vi "CloneManyMethods.vi"(1 "VIRefs":refnum<vi>[](array[refnum]), 5 "error in (no error)":errorcluster) -> (17 "Cancelled":bool, 19 "error out":errorcluster)   [LabVIEW 2020]
uses:
  <resource>/Framework/Providers/Open_GDS/SubVIs/GOOP_HelpButton.ctl
  <vilib>/picture/picture.llb/imagedata.ctl
  <vilib>/Utility/lvfile.llb/NI_FileType.lvlib
  <resource>/Framework/Providers/Open_GDS/ClassProviders/Provider_LvNativeClass/ClassWriterNative_class/ClassWriterNative.lvclass
panel:
  out "ProductPicture":picture
  in  "_CloneAndOpenVI":bool
  in  "_OverwirteTragetVIs":bool
  in  "_CloneMethodClasses":i32[](listbox) caption="Select which classes to clone the VI to"
  out "_ViPathAlreadyExists":bool=TRUE caption="This VI already exists"
  out "_CloneViName":string caption="Original VI Name"
  in  "_ClassOwner":u16(ring) caption="New VI Owner" items=["<Clone VIs to Selected Sibling Classes>", "<Clone VIs to Selected Classes>"]
  in  "_HelpCloneClass":T1
  in  "_Cancel":bool
  in  "_CloneVI":bool
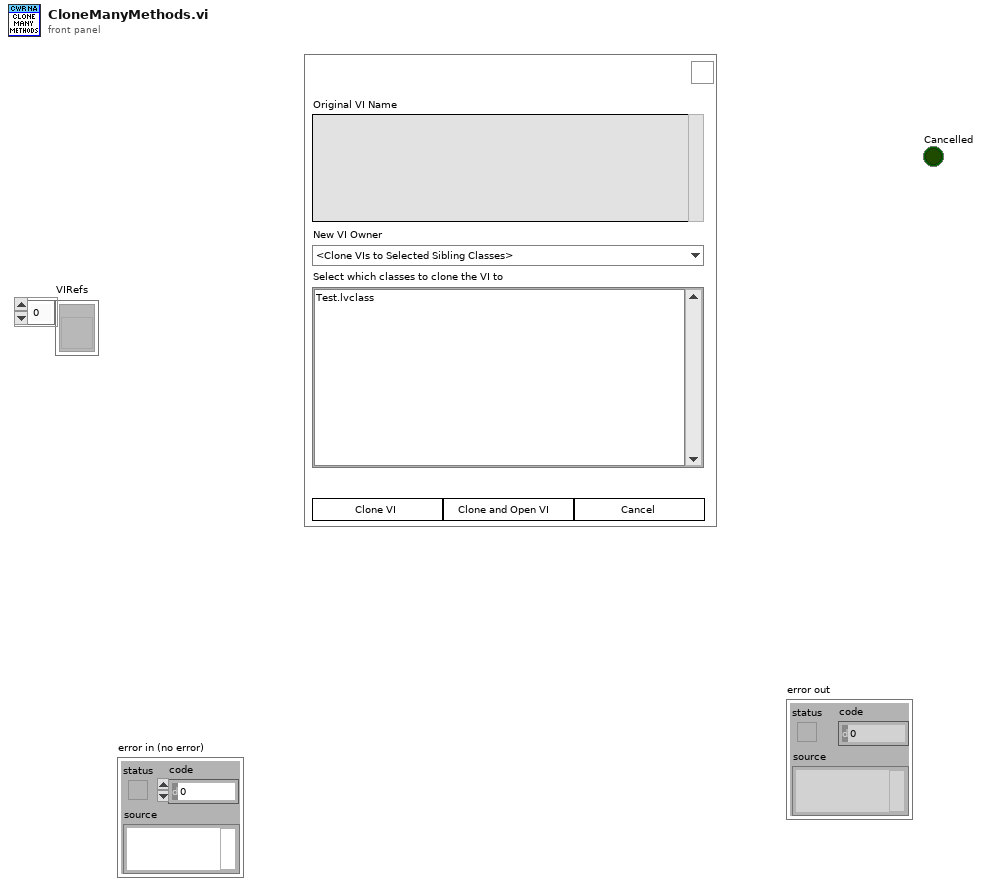
[diagram p1: front panel]
types:
  T1 = typedef "GOOP_HelpButton.ctl" = bool
  T2 = cluster{"Cancel":bool, "OrgVIPath":path, "Libs":refnum<vi>[], "SiblingClasses":refnum<vi>[], "ProjectFolder":path, "ViRelFromParent":path, "ManyClasses":bool, "OrgLibName":string, "AllClasses":refnum<vi>[], "OpenAfter":bool, "VIName":string[], "VIExt":string[], "AppRef":refnum<vi>, "VIOwner":refnum<vi>, "OrgViLibName":string, "OrgLibFolder":path, "OrgClassPath":path, "OrgClassPathMemberData":path, "FileBackups":string[], "CopyToTheseClasses":refnum<vi>[], "VIRef":refnum<vi>[], "OrgPath":path[], "Scope":enum32{"invalid scope", "public", "private", "protected", "community"}[], "NewViRefs":cluster{refnum<vi>[]}[], "NewVIPaths":path[]}
  T3 = enum32{"invalid scope", "public", "private", "protected", "community"}
  T4 = typedef "imagedata.ctl" = cluster{"image type":i32, "image depth":i32, "image":u8[], "mask":u8[], "colors":u32[], "Rectangle":cluster{"left":i16, "top":i16, "right":i16, "bottom":i16}}
  T5 = enum32{"invalid scope", "public", "private", "protected", "community"}[]
  T6 = typedef "GDSLvClass_IconSettingsType.ctl" = cluster{"Frame":u32, "Frame thickness":u8, "Header Background":u32, "Header Text":u32, "ColorPublic":u32, "ColorProtected":u32, "ColorPrivate":u32, "Body Text":u32, "ClassBodyIcon":string}
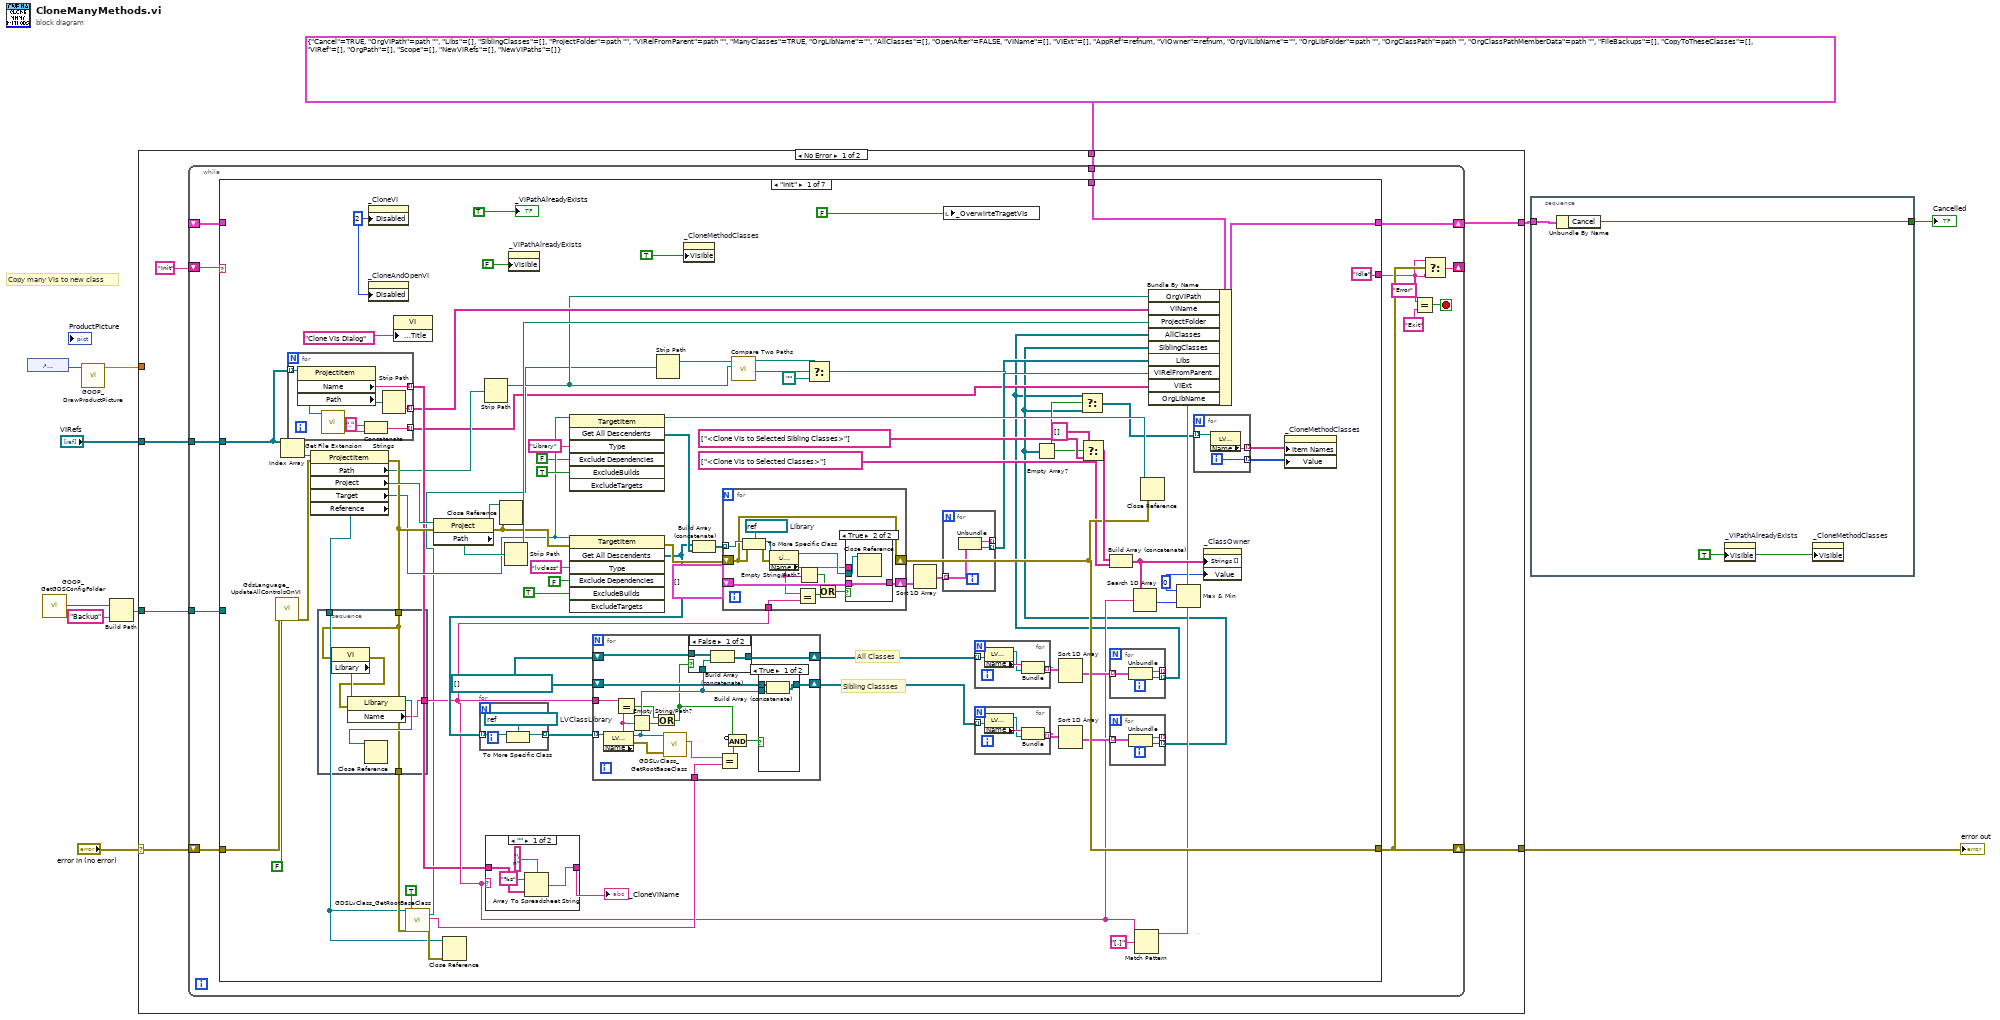
[diagram p0: block diagram]
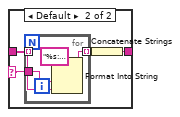
[diagram p2: hidden frame]
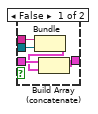
[diagram p5: hidden frame]
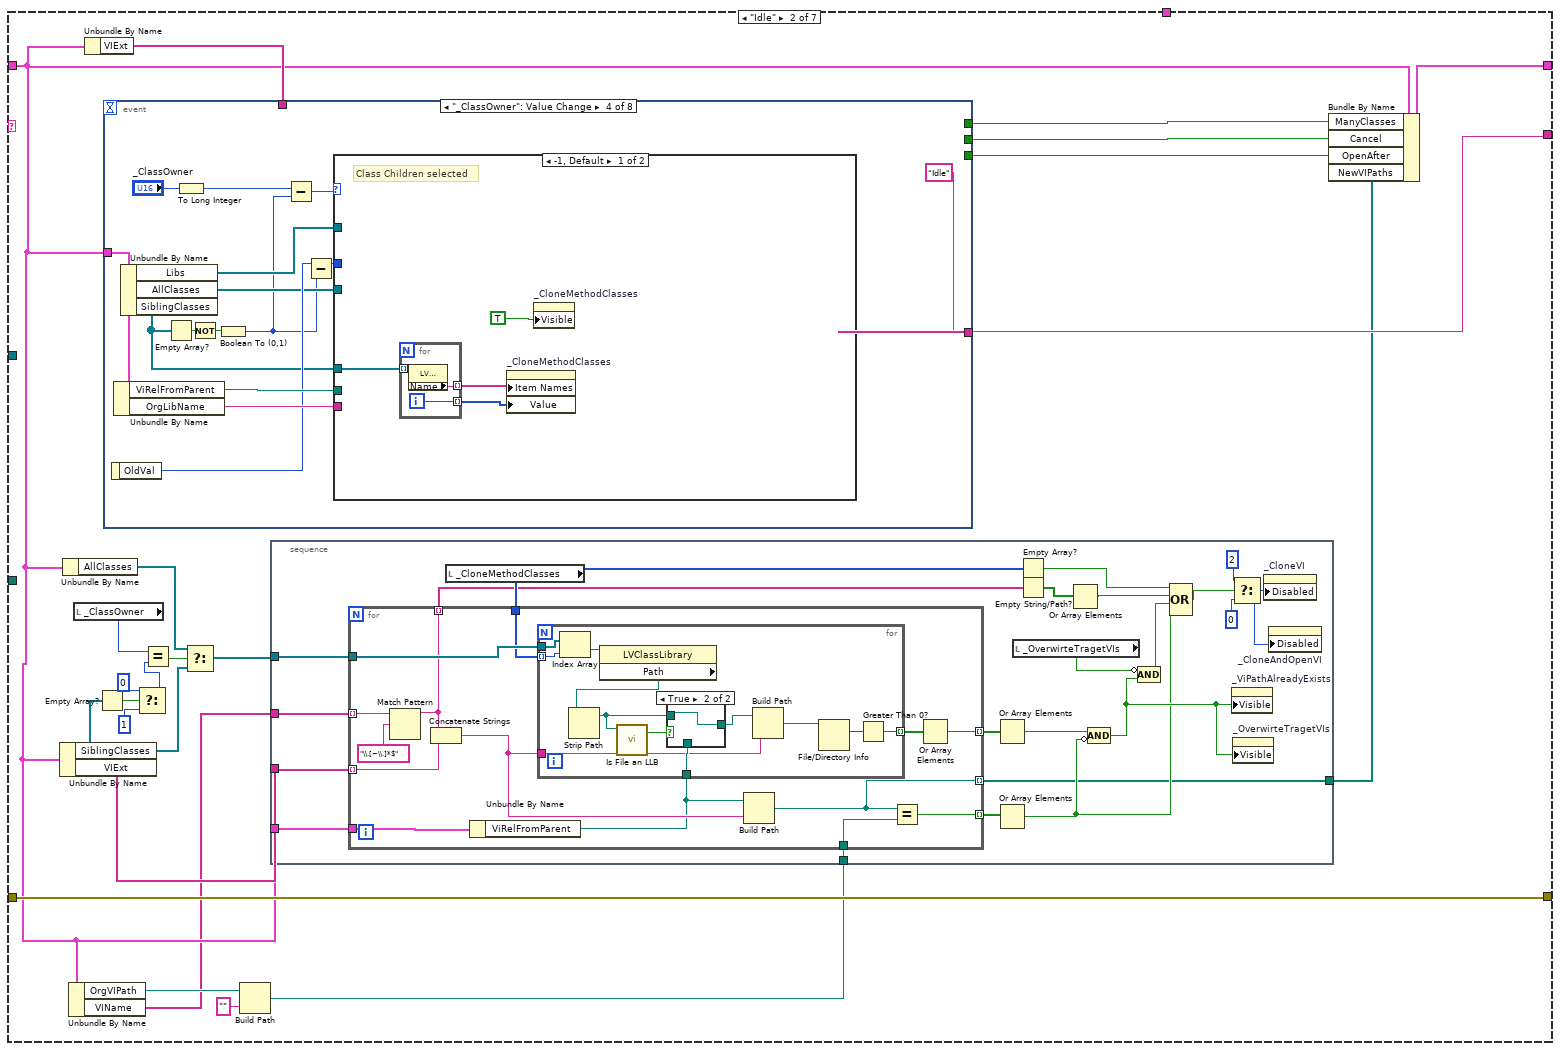
[diagram p6: hidden frame]
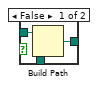
[diagram p7: hidden frame]
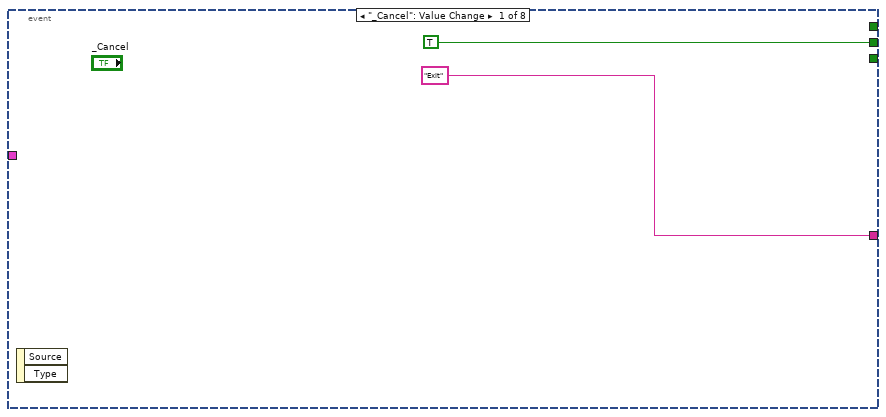
[diagram p8: hidden frame]
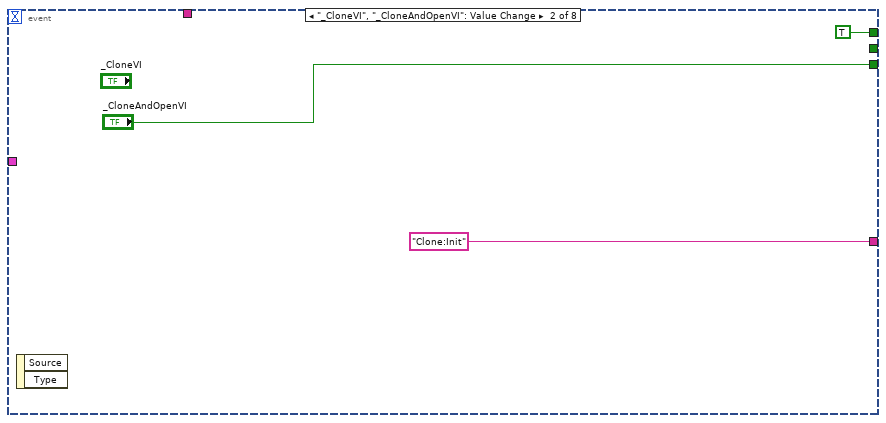
[diagram p9: hidden frame]
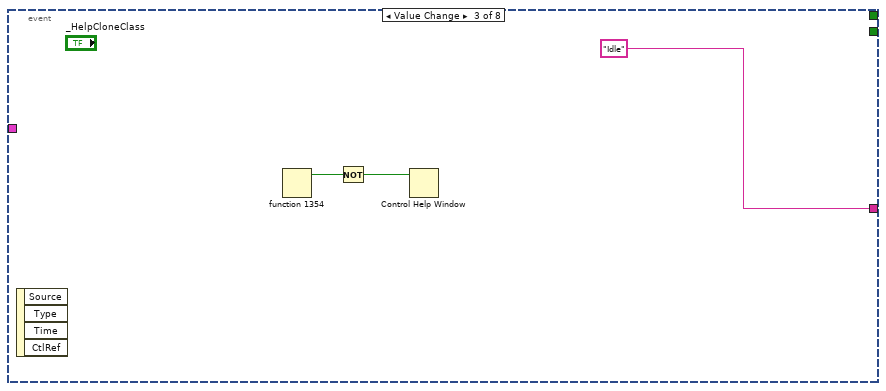
[diagram p10: hidden frame]
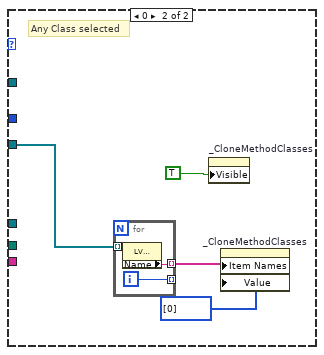
[diagram p11: hidden frame]
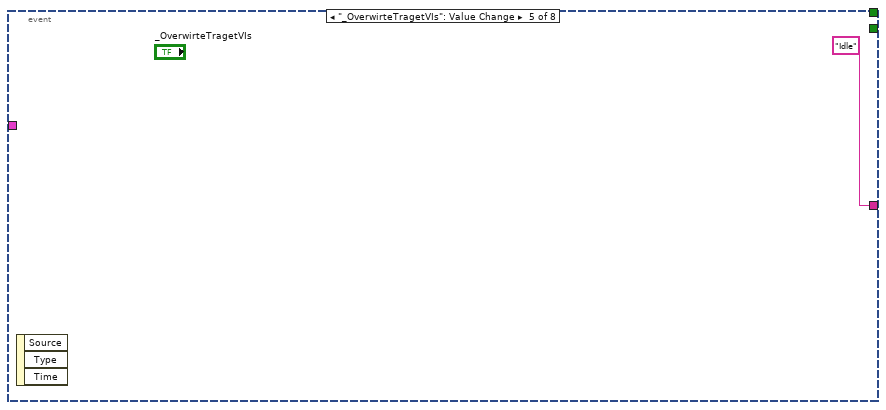
[diagram p12: hidden frame]
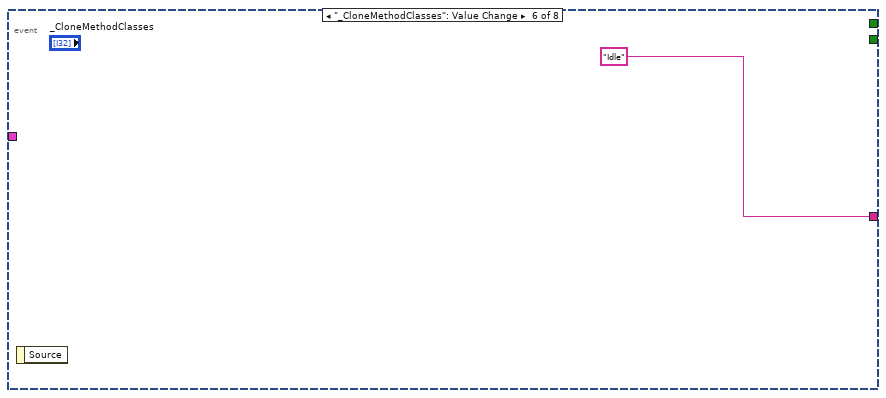
[diagram p13: hidden frame]
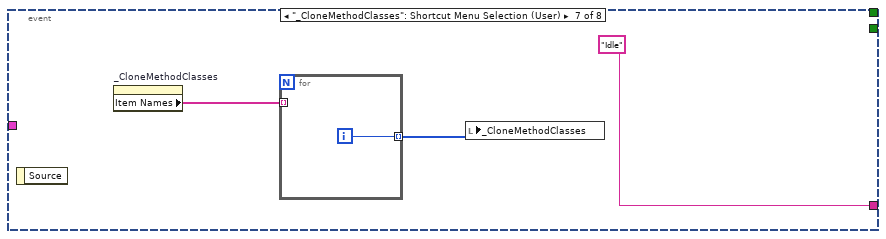
[diagram p14: hidden frame]
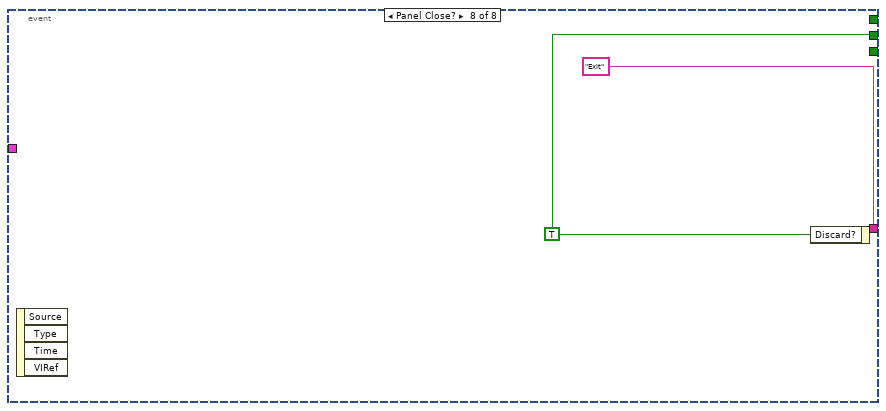
[diagram p15: hidden frame]
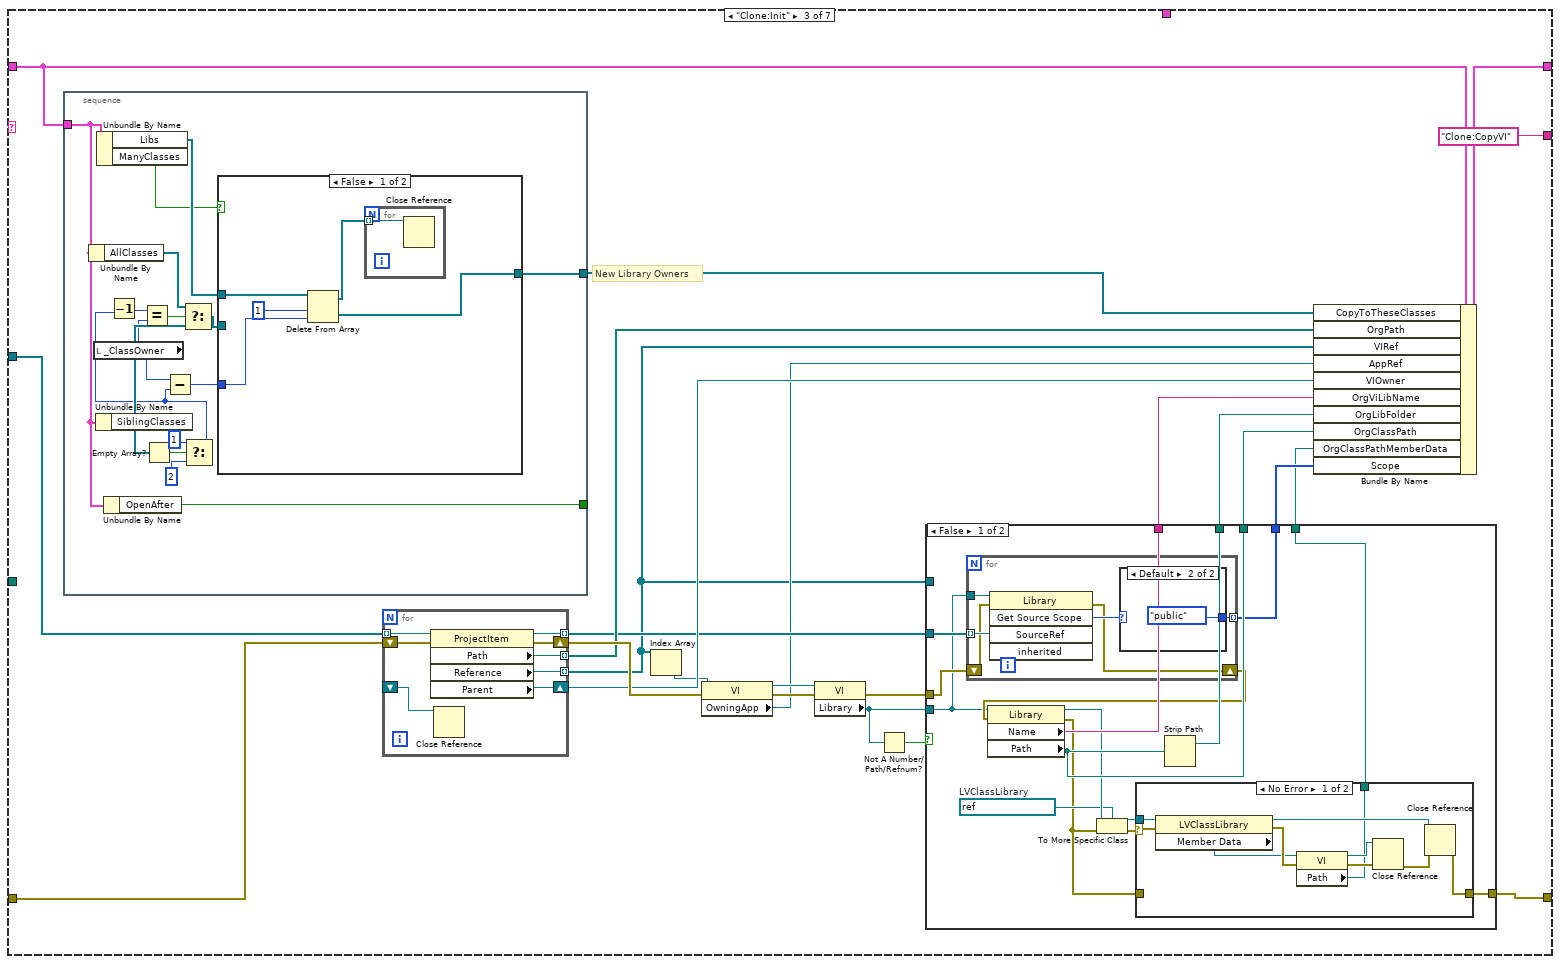
[diagram p16: hidden frame]
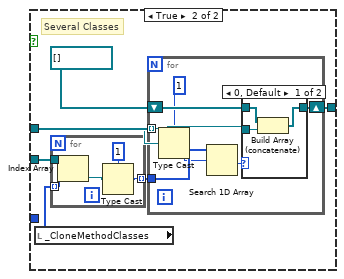
[diagram p17: hidden frame]
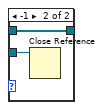
[diagram p18: hidden frame]
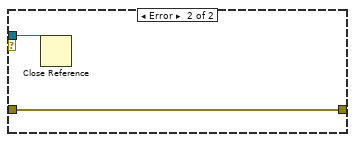
[diagram p20: hidden frame]
diagram:
  # "Copy many VIs to new class"
  n1 = control-ref of="ProductPicture"() -> (w2:refnum<vi>)
  n2 = call <resource>:"GOOP_GetGDSConfigFolder.vi"() -> ("GDSFolderPath"=w4:path)
  n3 = call <resource>:"GOOP_DrawProductPicture.vi"("ProductPictureControl"=w2) -> ("Zoom Factor"=w1:sgl)  [unwired: 10 in]
  n4 = Build Path(base path=w4, name or relative path="Backup") -> (appended path=w3:path)
  n5 = case shown="No Error" "error in (no error)" {
    selector: "error in (no error)" -> [w18 w819]
    tunnel: [w17 w819] -> w8
    tunnel: T2 {"Cancel"=TRUE, "OrgVIPath"=path "", "Libs"=[], "SiblingClasses"=[], "ProjectFolder"=path "", "ViRelFromParent"=path "", "ManyClasses"=TRUE, "OrgLibName"="", "AllClasses"=[], "OpenAfter"=FALSE, "VIName"=[], "VIExt"=[], "AppRef"=refnum, "VIOwner"=refnum, "OrgViLibName"="", "OrgLibFolder"=path "", "OrgClassPath"=path "", "OrgClassPathMemberData"=path "", "FileBackups"=[], "CopyToTheseClasses"=[], "VIRef"=[], "OrgPath"=[], "Scope"=[], "NewViRefs"=[], "NewVIPaths"=[]} ("output cluster") -> [w16 _]
    tunnel: "VIRefs" -> [w15 _]
    tunnel: [w14 _] -> w10
    tunnel: w3 -> [w12 _]
    tunnel: w1 -> [_ _]
    frame No Error {
      n6 = while {
        shift-right: [w25] -> w17
        shift-left: w18 -> [w31]
        shift-right: [w24] -> _
        shift-left: "Init" -> [w28]
        shift-right: [w29] -> w14
        shift-left: _ -> [w30]
        tunnel: w16 -> [w21]
        tunnel: w15 -> [w20]
        tunnel: w12 -> [w19]
        stop <- w26 stop-if-true
        n7 = case shown="\"Init\"" w28 {
          tunnel: w30 -> [_ w207 w326 w445 w620 w660 w769]
          tunnel: [w108 w222 w328 w447 w620 w660 w769] -> w29
          tunnel: w31 -> [w106 w224 w329 w449 w623 w663 w772]
          tunnel: [w79 w224 w330 w448 w622 w662 w771] -> w25
          tunnel: ["Idle" w223 "Clone:CopyVI" w446 "Clone:UpdateIcon" "Done" "Exit"] -> w23
          tunnel: w21 -> [w107 _ _ _ _ _ _]
          tunnel: w20 -> [w44 _ w324 _ _ _ _]
          tunnel: w19 -> [_ _ _ w443 _ _ w770]
          frame "Init" {
            w51 = 0 ("Text.Selection:Start")
            w73 = refnum<vi>[] []
            w71 = u8 2 ("Disabled")
            # "Sibling Classses"
            # "All Classes"
            n8 = call <resource>:"GdsLanguage_UpdateAllControlsOnVI.vi"("error in (no error)"=w106, "CreateLanguageFile(Use this to create a languageFile)"=FALSE) -> ("error out"=w52:errorcluster)  [unwired: 16 in, 1 out]
            n9 = Index Array(array=w44) -> (element=w45:refnum<vi>)  [unwired: 1 in]
            n10 = for {
              tunnel: w44 -> [w119] mode=indexing
              tunnel: [w118] -> w48 mode=indexing
              tunnel: [w117] -> w47 mode=indexing
              tunnel: [w113] -> w41 mode=indexing
              n11 = property class="ProjectItem"(reference=w119) -> ("Name"=w118:string, "Path"=w116:path)  [unwired: 1 in, 2 out]
              n12 = call <vilib>:"Get File Extension.vi"("file"=w116) -> ("lowercase file extension"=w114:string)  [unwired: 6 in, 4 out]
              n13 = Concatenate Strings("." ("string"), w114) -> (w113:string)
              n14 = Strip Path(path=w116) -> (name=w117:string)  [unwired: 1 out]
            }
            n15 = property class="ProjectItem"(reference=w45, error in=w52) -> (error out=w59:errorcluster, "Path"=w46:path, "Project"=w103:refnum<vi>, "Target"=w53:refnum<vi>, "Reference"=w54:refnum<vi>)  [unwired: 1 out]
            n16 = stacked-sequence {
              tunnel: w54 -> [w125]
              tunnel: w59 -> [w121]
              tunnel: [w120] -> w50
              tunnel: [w121] -> w58
              frame #0 {
                n17 = property class="VI"(reference=w125, error in=w121) -> (error out=w123:errorcluster, "Library"=w124:refnum<vi>)  [unwired: 1 out]
                n18 = property class="Library"(reference=w124, error in=w123) -> (reference out=w122:refnum<vi>, "Name"=w120:string)  [unwired: 1 out]
                n19 = Close Reference(reference=w122) -> ()  [unwired: 1 in, 1 out]
              }
            }
            n20 = property on="_CloneVI" class="Bool"("Disabled"=w71) -> ()  [unwired: 2 in, 2 out]
            n21 = property on="_CloneAndOpenVI" class="Bool"("Disabled"=w71) -> ()  [unwired: 2 in, 2 out]
            n22 = property class="VI"("Front Panel.Title"="Clone VIs Dialog" ("format string")) -> ()  [unwired: 2 in, 2 out]
            n23 = call <resource>:"GDSLvClass_GetRootBaseClass.vi"("ViRef/Path,LvClassRef/Path"=w54, "error in (no error)"=w58, "Don'tOpenReference"=TRUE) -> ("RootBaseClassPath"=w42:path, "ClassName"=w67:string, "error out"=w68:errorcluster)  [unwired: 10 in, 4 out]
            n24 = property class="Project"(reference=w103, error in=w59) -> (reference out=w80:refnum<vi>, error out=w81:errorcluster, "Path"=w83:path)
            n25 = Close Reference(reference=w54, error in (no error)=w68) -> ()  [unwired: 1 out]
            n26 = Strip Path(path=w46) -> (stripped path=w43:path)  [unwired: 1 out]
            n27 = case shown="\"\"" w50 {
              selector: w50 -> [_ w148]
              tunnel: w48 -> [w144 w150]
              tunnel: [w143 w147] -> w82
              frame "" {
                n28 = Array To Spreadsheet String(delimiter (Tab)="\n", array=w144, 3:"%s" ("format string")) -> (spreadsheet string=w143:string)
              }
              frame Default {
                n29 = for {
                  tunnel: w150 -> [w153] mode=indexing
                  tunnel: [w152] -> w149 mode=indexing
                  tunnel: w148 -> [w151]
                  n30 = Format Into String(format string="%s:%s\n", w151, w153) -> (resulting string=w152:string)  [unwired: 2 in, 1 out]
                }
                n31 = Concatenate Strings(w149) -> (w147:string)
              }
            }
            "_CloneViName" <- w82
            n32 = Close Reference(reference=w80, error in (no error)=w81) -> ()  [unwired: 1 out]
            n33 = Strip Path(path=w83) -> (stripped path=w88:path)  [unwired: 1 out]
            n34 = property on="_ViPathAlreadyExists" class="Bool (strict)"("Visible"=FALSE) -> ()  [unwired: 2 in, 2 out]
            n35 = invoke class="TargetItem" method="Get All Descendents"(reference=w53, "Type"="Library", "Exclude Dependencies"=FALSE ("ExcludeDependencies"), "ExcludeBuilds"=TRUE ("ExcludeDependencies")) -> (reference out=w78:refnum<vi>, "All Descendents"=w96:refnum<vi>[])  [unwired: 3 in, 5 out]
            n36 = invoke class="TargetItem" method="Get All Descendents"(reference=w53, error in=w81, "Type"="lvclass", "Exclude Dependencies"=FALSE ("ExcludeDependencies"), "ExcludeBuilds"=TRUE ("ExcludeDependencies")) -> (error out=w101:errorcluster, "All Descendents"=w94:refnum<vi>[])  [unwired: 2 in, 5 out]
            n37 = for {
              tunnel: w94 -> [w156] mode=indexing
              tunnel: [w155] -> w72 mode=indexing
              w157 = refnum<vi> refnum  # LVClassLibrary
              n38 = To More Specific Class(target class=w157, reference=w156) -> (specific class reference=w155:refnum<vi>)  [unwired: 1 in, 1 out]
            }
            n39 = for {
              tunnel: w72 -> [w173] mode=indexing
              tunnel: w67 -> [w165]
              shift-right: [w171] -> w60
              shift-left: w73 -> [w172]
              shift-right: [w169] -> w63
              shift-left: w73 -> [w170]
              tunnel: w50 -> [w168]
              n40 = property class="LVClassLibrary"(reference=w173) -> (reference out=w167:refnum<vi>, error out=w166:errorcluster, "Name"=w161:string)  [unwired: 1 in]
              n41 = Equal?(x=w168, y=w161) -> (x = y?=w159:bool)
              n42 = Empty String/Path?(string/path=w161) -> (empty?=w160:bool)
              n43 = Or(x=w159, y=w160) -> (x .or. y?=w158:bool)
              n44 = call <resource>:"GDSLvClass_GetRootBaseClass.vi"("ViRef/Path,LvClassRef/Path"=w167, "error in (no error)"=w166) -> ("ClassName"=w164:string)  [unwired: 11 in, 6 out]
              n45 = case shown="False" w158 {
                tunnel: w170 -> [w176 w177]
                tunnel: w167 -> [w175 _]
                tunnel: [w174 w177] -> w169
                frame False {
                  n46 = Build Array (concatenate)(w176, w175) -> (w174:refnum<vi>[])
                }
                frame True {
                }
              }
              n47 = Equal?(x=w164, y=w165) -> (x = y?=w163:bool)
              n48 = Compound Arithmetic op=AND(invert w158, w163) -> (w162:bool)
              n49 = case shown="True" w162 {
                tunnel: w172 -> [w180 w181]
                tunnel: w167 -> [w179 _]
                tunnel: [w178 w181] -> w171
                frame True {
                  n50 = Build Array (concatenate)(w180, w179) -> (w178:refnum<vi>[])
                }
                frame False {
                }
              }
            }
            n51 = Strip Path(path=w42) -> (stripped path=w89:path)  [unwired: 1 out]
            n52 = property on="_CloneMethodClasses" class="LstBox (strict)"("Visible"=TRUE) -> ()  [unwired: 2 in, 2 out]
            n53 = Build Array (concatenate)(w94, w96) -> (w95:refnum<vi>[])
            n54 = for {
              tunnel: w95 -> [w194] mode=indexing
              shift-right: [w189] -> w79
              shift-left: w101 -> [w189]
              shift-right: [w187] -> w56
              shift-left: cluster{"Name":string, refnum<vi>}[] [] -> [w188]
              tunnel: w50 -> [w186]
              w192 = refnum<vi> refnum  # Library
              n55 = To More Specific Class(target class=w192, reference=w194, error in=w189) -> (specific class reference=w193:refnum<vi>, error out=w191:errorcluster)
              n56 = property class="Library"(reference=w193, error in=w191) -> (reference out=w190:refnum<vi>, "Name"=w182:string)  [unwired: 1 out]
              n57 = Equal?(x=w182, y=w186) -> (x = y?=w184:bool)
              n58 = Empty String/Path?(string/path=w182) -> (empty?=w185:bool)
              n59 = Or(x=w185, y=w184) -> (x .or. y?=w183:bool)
              n60 = case shown="True" w183 {
                tunnel: w182 -> [w199 _]
                tunnel: w190 -> [w198 w200]
                tunnel: w188 -> [w197 w201]
                tunnel: [w195 w201] -> w187
                frame False {
                  n61 = Bundle("Name"=w199, w198) -> (w196:cluster{"Name":string, refnum<vi>})  [unwired: 1 in]
                  n62 = Build Array (concatenate)(w197, w196) -> (w195:cluster{"Name":string, refnum<vi>}[])
                }
                frame True {
                  n63 = Close Reference(reference=w200) -> ()  [unwired: 1 in, 1 out]
                }
              }
            }
            n64 = call <vilib>:"Compare Two Paths.vi"("Path 2"=w43, "Path 1"=w89) -> ("Path 2 Relative to Path 1?"=w87:bool, "Relative Path from 1 to 2"=w86:path)  [unwired: 6 in, 2 out]
            n65 = Select(t=w86, s=w87, f=path "") -> (s? t:f=w84:path)
            n66 = Sort 1D Array(array=w56) -> (sorted array=w70:cluster{"Name":string, refnum<vi>}[])
            n67 = for {
              tunnel: w70 -> [w142] mode=indexing
              tunnel: [w141] -> _ mode=indexing
              tunnel: [w140] -> w69 mode=indexing
              n68 = Unbundle(w142) -> ("Name"=w141:string, w140:refnum<vi>)
            }
            n69 = local write "_OverwirteTragetVIs"(FALSE ("Visible")) -> ()
            n70 = for {
              tunnel: w63 -> [w136] mode=indexing
              tunnel: [w137] -> w65 mode=indexing
              n71 = property class="LVClassLibrary"(reference=w136) -> (reference out=w138:refnum<vi>, "Name"=w139:string)  [unwired: 1 in, 1 out]
              n72 = Bundle("Name"=w139, w138) -> (w137:cluster{"Name":string, refnum<vi>})  [unwired: 1 in]
            }
            n73 = for {
              tunnel: w60 -> [w129] mode=indexing
              tunnel: [w130] -> w61 mode=indexing
              n74 = property class="LVClassLibrary"(reference=w129) -> (reference out=w131:refnum<vi>, "Name"=w132:string)  [unwired: 1 in, 1 out]
              n75 = Bundle("Name"=w132, w131) -> (w130:cluster{"Name":string, refnum<vi>})  [unwired: 1 in]
            }
            n76 = Sort 1D Array(array=w65) -> (sorted array=w64:cluster{"Name":string, refnum<vi>}[])
            n77 = Sort 1D Array(array=w61) -> (sorted array=w62:cluster{"Name":string, refnum<vi>}[])
            n78 = for {
              tunnel: w64 -> [w135] mode=indexing
              tunnel: [w134] -> _ mode=indexing
              tunnel: [w133] -> w35 mode=indexing
              n79 = Unbundle(w135) -> ("Name"=w134:string, w133:refnum<vi>)
            }
            n80 = for {
              tunnel: w62 -> [w128] mode=indexing
              tunnel: [w127] -> _ mode=indexing
              tunnel: [w126] -> w37 mode=indexing
              n81 = Unbundle(w128) -> ("Name"=w127:string, w126:refnum<vi>)
            }
            n82 = Empty Array?(array=w37) -> (empty?=w38:bool)
            n83 = Select(t=w35, s=w38, f=w37) -> (s? t:f=w36:refnum<vi>[])
            n84 = Select(t=string[] [], s=w38, f=string[] ["<Clone VIs to Selected Sibling Classes>"]) -> (s? t:f=w93:string[])
            n85 = Build Array (concatenate)(w93, string[] ["<Clone VIs to Selected Classes>"]) -> (w100:string[])
            n86 = Search 1D Array(1D array=w100, element=w50) -> (index of element=w99:i32)  [unwired: 1 in]
            n87 = Match Pattern(string=w50, regular expression="[.]") -> (before substring=w76:string)  [unwired: 1 in, 3 out]
            n88 = Close Reference(reference=w78, error in (no error)=w79) -> ()  [unwired: 1 out]
            n89 = Bundle By Name(cluster=w107, "OrgVIPath"=w43, "VIName"=w47, "ProjectFolder"=w88, "AllClasses"=w35, "SiblingClasses"=w37, "Libs"=w69, "ViRelFromParent"=w84, "VIExt"=w41, "OrgLibName"=w76) -> (w108:T2)
            n90 = Max & Min(x=w51, y=w99) -> ()  [unwired: 2 out]
            n91 = for {
              tunnel: [w112] -> w40 mode=indexing
              tunnel: w36 -> [w111] mode=indexing
              tunnel: [w110] -> w39 mode=indexing
              i -> [w110]
              n92 = property class="LVClassLibrary"(reference=w111) -> ("Name"=w112:string)  [unwired: 1 in, 2 out]
            }
            n93 = property on="_ClassOwner" class="Ring (strict)"("Strings []"=w100, "Value"=w51) -> ()  [unwired: 2 in, 2 out]
            n94 = property on="_CloneMethodClasses" class="LstBox (strict)"("Item Names"=w40, "Value"=w39) -> ()  [unwired: 2 in, 2 out]
            "_ViPathAlreadyExists" <- TRUE ("Visible")
          }
          frame "Idle" {
            n95 = Unbundle By Name(w207) -> ("SiblingClasses"=w213:refnum<vi>[], "VIExt"=w219:string[])
            n96 = Unbundle By Name(w207) -> ("AllClasses"=w216:refnum<vi>[])
            n97 = Unbundle By Name(w207) -> ("OrgVIPath"=w206:path, "VIName"=w204:string[])
            n98 = local read "_ClassOwner"() -> (w211:u16)
            n99 = Unbundle By Name(w207) -> ("VIExt"=w220:string[])
            n100 = Empty Array?(array=w213) -> (empty?=w214:bool)
            n101 = event shown="[3] \"_ClassOwner\": Value Change" {
              selector: _ -> [_ _ _ _ _ _ _ _]
              dyn-events: _ -> [_ _ _ _ _ _ _ _]
              timeout: _ -> [_ _ _ _ _ _ _ _]
              tunnel: ["Exit" "Clone:Init" "Idle" "Idle" "Idle" "Idle" "Idle" "Exit"] -> w223
              tunnel: [TRUE _ _ _ _ _ _ w321] -> w221
              tunnel: w207 -> [_ _ _ w296 _ _ _ _]
              tunnel: w220 -> [_ _ _ _ _ _ _ _]
              tunnel: [_ TRUE ("Visible") _ _ _ _ _ _] -> w218
              tunnel: [_ "_CloneAndOpenVI" _ _ _ _ _ _] -> w208
              event "_Cancel": Value Change {
                n102 = event-data() -> ()  [unwired: 1 in, 2 out]
              }
              event "_CloneVI", "_CloneAndOpenVI": Value Change {
                n103 = event-data() -> ()  [unwired: 1 in, 2 out]
              }
              event Value Change {
                n104 = event-data() -> ()  [unwired: 1 in, 4 out]
                n105 = fn#1354() -> (1:w284:bool)  [unwired: 1 out]
                n106 = Not(x=w284) -> (.not. x?=w283:bool)
                n107 = Control Help Window(1:w283) -> ()  [unwired: 1 in]
              }
              event "_ClassOwner": Value Change {
                n108 = event-data() -> ("OldVal"=w291:u16)  [unwired: 1 in]
                n109 = Unbundle By Name(w296) -> ("ViRelFromParent"=w295:path, "OrgLibName"=w292:string)
                n110 = Unbundle By Name(w296) -> ("Libs"=w297:refnum<vi>[], "AllClasses"=w288:refnum<vi>[], "SiblingClasses"=w289:refnum<vi>[])
                n111 = Empty Array?(array=w289) -> (empty?=w298:bool)
                n112 = To Long Integer(number="_ClassOwner") -> (32bit integer=w290:i32)
                n113 = Not(x=w298) -> (.not. x?=w293:bool)
                n114 = Boolean To (0,1)(Boolean=w293) -> (0, 1=w285:i16)
                n115 = Subtract(x=w290, y=w285) -> (x-y=w287:i32)
                n116 = Subtract(x=w291, y=w285) -> (x-y=w286:u16)
                n117 = case shown="-1, Default" w287 {
                  tunnel: w297 -> [_ _]
                  tunnel: w295 -> [_ _]
                  tunnel: w292 -> [_ _]
                  tunnel: w286 -> [_ _]
                  tunnel: w289 -> [w302 _]
                  tunnel: w288 -> [_ w308]
                  frame -1, Default {
                    # "Class Children selected"
                    n118 = for {
                      tunnel: [w306] -> w301 mode=indexing
                      tunnel: w302 -> [w305] mode=indexing
                      tunnel: [w304] -> w300 mode=indexing
                      i -> [w304]
                      n119 = property class="LVClassLibrary"(reference=w305) -> ("Name"=w306:string)  [unwired: 1 in, 2 out]
                    }
                    n120 = property on="_CloneMethodClasses" class="LstBox (strict)"("Item Names"=w301, "Value"=w300) -> ()  [unwired: 2 in, 2 out]
                    n121 = property on="_CloneMethodClasses" class="LstBox (strict)"("Visible"=TRUE) -> ()  [unwired: 2 in, 2 out]
                  }
                  frame 0 {
                    # "Any Class selected"
                    n122 = for {
                      tunnel: [w313] -> w309 mode=indexing
                      tunnel: w308 -> [w312] mode=indexing
                      tunnel: [w311] -> _ mode=indexing
                      i -> [w311]
                      n123 = property class="LVClassLibrary"(reference=w312) -> ("Name"=w313:string)  [unwired: 1 in, 2 out]
                    }
                    n124 = property on="_CloneMethodClasses" class="LstBox (strict)"("Visible"=TRUE) -> ()  [unwired: 2 in, 2 out]
                    n125 = property on="_CloneMethodClasses" class="LstBox (strict)"("Item Names"=w309, "Value"=i32[] [0] ("_CloneMethodClasses")) -> ()  [unwired: 2 in, 2 out]
                  }
                }
              }
              event "_OverwirteTragetVIs": Value Change {
                n126 = event-data() -> ()  [unwired: 1 in, 3 out]
              }
              event "_CloneMethodClasses": Value Change {
                n127 = event-data() -> ()  [unwired: 1 in, 1 out]
              }
              event "_CloneMethodClasses": Shortcut Menu Selection (User) {
                n128 = event-data() -> ()  [unwired: 1 in, 1 out]
                n129 = property on="_CloneMethodClasses" class="LstBox (strict)"() -> ("Item Names"=w316:string[])  [unwired: 2 in, 2 out]
                n130 = for {
                  tunnel: [w319] -> w318 mode=indexing
                  tunnel: w316 -> [_] mode=indexing
                  i -> [w319]
                }
                n131 = local write "_CloneMethodClasses"(w318) -> ()
              }
              event Panel Close? {
                w321 = TRUE ("Discard?")
                n132 = event-data() -> ()  [unwired: 1 in, 4 out]
                n133 = event-data("Discard?"=w321) -> ()  [unwired: 1 in, 1 out]
              }
            }
            n134 = Select(t=u16 0 ("x"), s=w214, f=u16 1 ("x")) -> (s? t:f=w210:u16)
            n135 = Equal?(x=w211, y=w210) -> (x = y?=w212:bool)
            n136 = Select(t=w216, s=w212, f=w213) -> (s? t:f=w217:refnum<vi>[])
            n137 = Build Path(base path=w206, name or relative path="") -> (appended path=w203:path)
            n138 = stacked-sequence {
              tunnel: w219 -> [w244]
              tunnel: w217 -> [w243]
              tunnel: w207 -> [w242]
              tunnel: w204 -> [w233]
              tunnel: w203 -> [w230]
              tunnel: [w225] -> w202
              frame #0 {
                n139 = local read "_CloneMethodClasses"() -> (w238:i32[])
                n140 = for {
                  tunnel: w244 -> [w258] mode=indexing
                  tunnel: w243 -> [w257]
                  tunnel: w242 -> [w256]
                  tunnel: w238 -> [w253]
                  tunnel: [w252] -> w234 mode=indexing
                  tunnel: w233 -> [w251] mode=indexing
                  tunnel: [w250] -> w232 mode=indexing
                  tunnel: w230 -> [w249]
                  tunnel: [w248] -> w229 mode=indexing
                  tunnel: [w247] -> w225 mode=indexing
                  n141 = Match Pattern(string=w251, regular expression="\\.[~\\.]*$") -> (before substring=w250:string)  [unwired: 1 in, 3 out]
                  n142 = Concatenate Strings(w250, w258) -> (w260:string)
                  n143 = Unbundle By Name(w256) -> ("ViRelFromParent"=w254:path)
                  n144 = for {
                    tunnel: w257 -> [w272]
                    tunnel: w253 -> [w271] mode=indexing
                    tunnel: w254 -> [w268]
                    tunnel: w260 -> [w266]
                    tunnel: [w263] -> w255 mode=indexing
                    n145 = Index Array(array=w272, index=w271) -> (element=w270:refnum<vi>)
                    n146 = property class="LVClassLibrary"(reference=w270) -> ("Path"=w269:path)  [unwired: 1 in, 2 out]
                    n147 = Strip Path(path=w269) -> (stripped path=w262:path)  [unwired: 1 out]
                    n148 = call <vilib>:"Is File an LLB.vi"("path"=w262) -> ("Is LLB?"=w261:bool)  [unwired: 9 in, 1 out]
                    n149 = case shown="True" w261 {
                      tunnel: w268 -> [w275 _]
                      tunnel: [w274 w276] -> w267
                      tunnel: w262 -> [w273 w276]
                      frame False {
                        n150 = Build Path(base path=w273, name or relative path=w275) -> (appended path=w274:path)
                      }
                      frame True {
                      }
                    }
                    n151 = Build Path(base path=w267, name or relative path=w266) -> (appended path=w264:path)
                    n152 = File/Directory Info(path=w264) -> (size=w265:i64)  [unwired: 1 in, 6 out]
                    n153 = Greater Than 0?(x=w265) -> (x > 0?=w263:bool)
                  }
                  n154 = Build Path(base path=w254, name or relative path=w260) -> (appended path=w247:path)
                  n155 = Equal?(x=w247, y=w249) -> (x = y?=w248:bool)
                  n156 = Or Array Elements(Boolean array=w255) -> (logical OR=w252:bool)
                }
                n157 = Or Array Elements(Boolean array=w234) -> (logical OR=w231:bool)
                n158 = Or Array Elements(Boolean array=w229) -> (logical OR=w228:bool)
                n159 = local read "_OverwirteTragetVIs"() -> (w236:bool)
                n160 = Empty Array?(array=w238) -> (empty?=w237:bool)
                n161 = Empty String/Path?(string/path=w232) -> (empty?=w227:bool[])
                n162 = Or Array Elements(Boolean array=w227) -> (logical OR=w226:bool)
                n163 = Compound Arithmetic op=AND(w231, invert w228) -> (w240:bool)
                n164 = Compound Arithmetic op=AND(invert w236, w240) -> (w235:bool)
                n165 = Compound Arithmetic op=OR(w237, w226, w235, w228) -> (w241:bool)
                n166 = Select(t=u8 2, s=w241, f=u8 0 ("Disabled")) -> (s? t:f=w239:u8)
                n167 = property on="_ViPathAlreadyExists" class="Bool (strict)"("Visible"=w240) -> ()  [unwired: 2 in, 2 out]
                n168 = property on="_OverwirteTragetVIs" class="Bool (strict)"("Visible"=w240) -> ()  [unwired: 2 in, 2 out]
                n169 = property on="_CloneVI" class="Bool"("Disabled"=w239) -> ()  [unwired: 2 in, 2 out]
                n170 = property on="_CloneAndOpenVI" class="Bool"("Disabled"=w239) -> ()  [unwired: 2 in, 2 out]
              }
            }
            n171 = Bundle By Name(cluster=w207, "ManyClasses"=w218, "Cancel"=w221, "OpenAfter"=w208, "NewVIPaths"=w202) -> (w222:T2)
          }
          frame "Clone:Init" {
            # "New Library Owners"
            n172 = stacked-sequence {
              tunnel: w326 -> [w355]
              tunnel: [w368] -> w325
              tunnel: [w354] -> _
              frame #0 {
                n173 = Unbundle By Name(w355) -> ("AllClasses"=w360:refnum<vi>[])
                n174 = local read "_ClassOwner"() -> (w359:u16)
                n175 = Unbundle By Name(w355) -> ("SiblingClasses"=w362:refnum<vi>[])
                n176 = Unbundle By Name(w355) -> ("Libs"=w369:refnum<vi>[], "ManyClasses"=w363:bool)
                n177 = Unbundle By Name(w355) -> ("OpenAfter"=w354:bool)
                n178 = Empty Array?(array=w362) -> (empty?=w367:bool)
                n179 = Select(t=u16 1 ("x"), s=w367, f=u16 2 ("x")) -> (s? t:f=w356:u16)
                n180 = Decrement(x=w356) -> (x-1=w357:u16)
                n181 = Equal?(x=w357, y=w359) -> (x = y?=w358:bool)
                n182 = Subtract(x=w359, y=w356) -> (x-y=w364:u16)
                n183 = Select(t=w360, s=w358, f=w362) -> (s? t:f=w361:refnum<vi>[])
                n184 = case shown="False" w363 {
                  tunnel: w369 -> [w374 w381]
                  tunnel: [w371 w379] -> w368
                  tunnel: w364 -> [w373 _]
                  tunnel: w361 -> [_ w378]
                  frame False {
                    n185 = Delete From Array(array=w374, length=1, index=w373) -> (deleted portion=w371:refnum<vi>[], array with subset deleted=w370:refnum<vi>[])
                    n186 = for {
                      tunnel: w370 -> [w375] mode=indexing
                      n187 = Close Reference(reference=w375) -> ()  [unwired: 1 in, 1 out]
                    }
                  }
                  frame True {
                    # "Several Classes"
                    n188 = local read "_CloneMethodClasses"() -> (w377:i32[])
                    n189 = for {
                      tunnel: w378 -> [w386]
                      tunnel: w377 -> [w385] mode=indexing
                      tunnel: [w383] -> w376 mode=indexing
                      n190 = Index Array(array=w386, index=w385) -> (element=w384:refnum<vi>)
                      n191 = Type Cast(type=u32 1 ("x"), x=w384) -> (*(type *) &x=w383:u32)
                    }
                    n192 = for {
                      tunnel: w381 -> [w389] mode=indexing
                      shift-right: [w392] -> w379
                      shift-left: refnum<vi>[] [] -> [w393]
                      tunnel: w376 -> [w390]
                      n193 = Type Cast(type=u32 1 ("x"), x=w389) -> (*(type *) &x=w387:u32)
                      n194 = Search 1D Array(1D array=w390, element=w387) -> (index of element=w391:i32)  [unwired: 1 in]
                      n195 = case shown="0, Default" w391 {
                        tunnel: w389 -> [w396 w397]
                        tunnel: w393 -> [w395 w398]
                        tunnel: [w394 w398] -> w392
                        frame 0, Default {
                          n196 = Build Array (concatenate)(w395, w396) -> (w394:refnum<vi>[])
                        }
                        frame -1 {
                          n197 = Close Reference(reference=w397) -> ()  [unwired: 1 in, 1 out]
                        }
                      }
                    }
                  }
                }
              }
            }
            n198 = for {
              tunnel: [w353] -> w322 mode=indexing
              tunnel: [w350] -> w339 mode=indexing
              tunnel: [w349] -> w337 mode=indexing
              tunnel: w324 -> [w347] mode=indexing
              shift-right: [w352] -> w345
              shift-left: w329 -> [w348]
              shift-right: [w351] -> w344
              shift-left: _ -> [w346]
              n199 = property class="ProjectItem"(reference=w347, error in=w348) -> (reference out=w349:refnum<vi>, error out=w352:errorcluster, "Path"=w350:path, "Reference"=w353:refnum<vi>, "Parent"=w351:refnum<vi>)
              n200 = Close Reference(reference=w346) -> ()  [unwired: 1 in, 1 out]
            }
            n201 = Index Array(array=w322) -> (element=w323:refnum<vi>)  [unwired: 1 in]
            n202 = property class="VI"(reference=w323, error in=w345) -> (reference out=w343:refnum<vi>, error out=w342:errorcluster, "OwningApp"=w331:refnum<vi>)
            n203 = property class="VI"(reference=w343, error in=w342) -> (error out=w335:errorcluster, "Library"=w334:refnum<vi>)  [unwired: 1 out]
            n204 = Not A Number/Path/Refnum?(number/path/refnum=w334) -> (NaN/Path/Refnum?=w332:bool)
            n205 = case shown="False" w332 {
              tunnel: [w413 _] -> w341
              tunnel: [w412 _] -> w340
              tunnel: [w411 _] -> w338
              tunnel: [w410 w438] -> w330
              tunnel: w337 -> [w404 _]
              tunnel: [w403 w434] -> w336
              tunnel: w335 -> [w402 w438]
              tunnel: w334 -> [w399 _]
              tunnel: [w400 _] -> w333
              tunnel: w322 -> [_ w437]
              frame False {
                w408 = refnum<vi> refnum  # LVClassLibrary
                n206 = for {
                  tunnel: w404 -> [w419] mode=indexing
                  tunnel: [w417] -> w403 mode=indexing
                  tunnel: w399 -> [w415]
                  shift-right: [w416] -> w401
                  shift-left: w402 -> [w414]
                  n207 = invoke class="Library" method="Get Source Scope"(reference=w415, error in=w414, "SourceRef"=w419) -> (error out=w416:errorcluster, "GetSourceScope"=w418:T3)  [unwired: 2 in, 3 out]
                  n208 = case shown="Default" w418 {
                    selector: w418 -> [w420 _]
                    tunnel: [w420 T3."public" ("GetSourceScope")] -> w417
                    frame "private", "protected" {
                    }
                    frame Default {
                    }
                  }
                }
                n209 = property class="Library"(reference=w399, error in=w401) -> (reference out=w409:refnum<vi>, error out=w406:errorcluster, "Name"=w413:string, "Path"=w411:path)
                n210 = To More Specific Class(target class=w408, reference=w409, error in=w406) -> (specific class reference=w405:refnum<vi>, error out=w407:errorcluster)
                n211 = case shown="No Error" w407 {
                  selector: w407 -> [w424 _]
                  tunnel: [w425 w433] -> w410
                  tunnel: w406 -> [_ w433]
                  tunnel: [w423 _] -> w400
                  tunnel: w405 -> [w422 w432]
                  frame No Error {
                    n212 = property class="LVClassLibrary"(reference=w422, error in=w424) -> (reference out=w427:refnum<vi>, error out=w431:errorcluster, "Member Data"=w430:refnum<vi>)
                    n213 = property class="VI"(reference=w430, error in=w431) -> (reference out=w428:refnum<vi>, error out=w429:errorcluster, "Path"=w423:path)
                    n214 = Close Reference(reference=w428, error in (no error)=w429) -> (error out=w426:errorcluster)
                    n215 = Close Reference(reference=w427, error in (no error)=w426) -> (error out=w425:errorcluster)
                  }
                  frame Error {
                    n216 = Close Reference(reference=w432) -> ()  [unwired: 1 in, 1 out]
                  }
                }
                n217 = Strip Path(path=w411) -> (stripped path=w412:path)  [unwired: 1 out]
              }
              frame True {
                n218 = Array Size(array=w437) -> (size(s)=w436:i32)
                n219 = Initialize Array(T3."public" ("GetSourceScope"), w436) -> (w434:T5)
              }
            }
            n220 = Bundle By Name(cluster=w326, "CopyToTheseClasses"=w325, "OrgPath"=w339, "VIRef"=w322, "AppRef"=w331, "VIOwner"=w344, "OrgViLibName"=w341, "OrgLibFolder"=w340, "OrgClassPath"=w338, "OrgClassPathMemberData"=w333, "Scope"=w336) -> (w328:T2)
          }
          frame "Clone:CopyVI" {
            n221 = Unbundle By Name(w445) -> ("NewVIPaths"=w440:path[], "CopyToTheseClasses"=w444:refnum<vi>[])
            n222 = Unbundle By Name(w445) -> ("AppRef"=w455:refnum<vi>, "VIRef"=w442:refnum<vi>[], "Scope"=w451:T5, "VIOwner"=w454:refnum<vi>, "OrgPath"=w453:path[], "OrgLibFolder"=w439:path, "OrgViLibName"=w452:string)
            n223 = Empty Array?(array=w444) -> (empty?=w456:bool)
            n224 = case shown="False" w456 {
              tunnel: w444 -> [w472 _]
              tunnel: w442 -> [w471 w567]
              tunnel: w440 -> [w470 w564]
              tunnel: w449 -> [w469 w565]
              tunnel: [w468 w562] -> w448
              tunnel: ["Clone:NewLibraryReplaceControlsAndVIs" w560] -> w446
              tunnel: w455 -> [w467 w566]
              tunnel: [w460 _] -> w441
              tunnel: w454 -> [_ w561]
              tunnel: w453 -> [w458 w563]
              tunnel: w452 -> [w466 _]
              tunnel: w451 -> [w465 _]
              tunnel: w443 -> [w464 _]
              tunnel: [w462 _] -> w450
              tunnel: w439 -> [w457 _]
              frame False {
                (unwired) "Clone:UpdateIcon"
                # "A library owns the VI(s)"
                n225 = for {
                  tunnel: w472 -> [w490]
                  tunnel: w471 -> [w489] mode=indexing
                  tunnel: w470 -> [w476] mode=indexing
                  tunnel: w467 -> [w486]
                  tunnel: w466 -> [w485]
                  tunnel: [w483] -> w461 mode=indexing
                  tunnel: w465 -> [w482] mode=indexing
                  tunnel: w464 -> [w481]
                  shift-right: [w479] -> w462
                  shift-left: string[] [] -> [w480]
                  shift-right: [w487] -> w468
                  shift-left: w469 -> [w488]
                  tunnel: [w477] -> w460 mode=indexing
                  tunnel: w458 -> [w474] mode=indexing
                  tunnel: w457 -> [w475]
                  # "For every VI to Clone"
                  n226 = call <vilib>:"Compare Two Paths.vi"("Path 2"=w474, "Path 1"=w475) -> ("Relative Path from 1 to 2"=w473:path)  [unwired: 6 in, 3 out]
                  n227 = for {
                    tunnel: w490 -> [w507] mode=indexing
                    tunnel: w489 -> [w495]
                    tunnel: w476 -> [w517]
                    shift-right: [w508] -> w487
                    shift-left: w488 -> [w516]
                    tunnel: w486 -> [w513]
                    tunnel: [w510] -> w478 mode=indexing
                    tunnel: w485 -> [w496]
                    tunnel: [w509] -> w484 mode=indexing
                    tunnel: w482 -> [w506]
                    tunnel: w481 -> [w505]
                    shift-right: [w502] -> w479
                    shift-left: w480 -> [w503]
                    tunnel: w473 -> [w491]
                    # "For every Class to clone this VI to"
                    n228 = property class="Library"(reference=w507) -> ("Path"=w493:path)  [unwired: 1 in, 2 out]
                    n229 = Strip Path(path=w493) -> (stripped path=w492:path)  [unwired: 1 out]
                    n230 = disable-structure shown="Enabled" {
                      disable-tunnel: w517 -> [w521 _]
                      disable-tunnel: [w520 w529] -> w498
                      disable-tunnel: w492 -> [w519 w531]
                      disable-tunnel: w491 -> [_ w530]
                      frame Disabled {
                        n231 = call <vilib>:"Is File an LLB.vi"("path"=w519) -> ("Is LLB?"=w518:bool)  [unwired: 9 in, 1 out]
                        n232 = case shown="False" w518 {
                          tunnel: w521 -> [w524 w526]
                          tunnel: w519 -> [w523 w527]
                          tunnel: [w522 w528] -> w520
                          frame False {
                            n233 = Build Path(base path=w523, name or relative path=w524) -> (appended path=w522:path)
                          }
                          frame True {
                            n234 = Strip Path(path=w526) -> (name=w525:string)  [unwired: 1 out]
                            n235 = Build Path(base path=w527, name or relative path=w525) -> (appended path=w528:path)
                          }
                        }
                      }
                      frame Enabled {
                        n236 = Build Path(base path=w531, name or relative path=w530) -> (appended path=w529:path)
                      }
                    }
                    n237 = stacked-sequence {
                      tunnel: w498 -> [w553]
                      tunnel: [w553] -> w497
                      frame #0 {
                        n238 = Strip Path(path=w553) -> (stripped path=w554:path)  [unwired: 1 out]
                        n239 = call <resource>:"GDSFile_CreateFolders.vi"("Path"=w554, "Promt if folder\ndoes not exists?"=FALSE ("Promt if folder\ndoes not exists?")) -> ()  [unwired: 13 in, 5 out]
                      }
                    }
                    n240 = call <resource>:"GDSFile_SaveViCopy.vi"("BackupFolder"=w505, "error in"=w516, "OverWirite(False)"=TRUE, "NewCopyPath"=w497, "VIRef"=w495) -> ("error out"=w514:errorcluster, "BackupFileName"=w501:path)  [unwired: 4 in, 1 out]
                    n241 = Strip Path(path=w501) -> (name=w500:string)  [unwired: 1 out]
                    n242 = Empty String/Path?(string/path=w501) -> (empty?=w504:bool)
                    n243 = Open VI Reference(application reference (local)=w513, vi path=w497, options=2, error in (no error)=w514) -> (vi reference=w510:refnum<vi>, error out=w511:errorcluster)  [unwired: 2 in]
                    n244 = case shown="False" FALSE {
                      tunnel: [w542 w552] -> w512
                      tunnel: w511 -> [w541 w551]
                      tunnel: w510 -> [w540 _]
                      tunnel: [w539 w551] -> w508
                      tunnel: w507 -> [w538 _]
                      tunnel: w506 -> [w534 _]
                      tunnel: w496 -> [_ w552]
                      frame False {
                        n245 = property class="VI"(reference=w540, error in=w541) -> (error out=w547:errorcluster, "Path"=w548:path)  [unwired: 1 out]
                        n246 = call <resource>:"GDSLvClass_GetLibraryItemFromPath.vi"("Library Refnum In"=w538, "VINames"=w548, "error in (no error)"=w547) -> ("Item Refnum Out"=w545:refnum<vi>, "error out"=w546:errorcluster)  [unwired: 15 in]
                        n247 = invoke class="ProjectItem" method="AddFile"(reference=w545, error in=w546, "Path"=w548) -> (error out=w533:errorcluster, "AddFile"=w535:refnum<vi>)  [unwired: 1 in, 2 out]
                        n248 = stacked-sequence {
                          tunnel: [w549] -> w532
                          tunnel: w533 -> [w549]
                          frame #0 {
                            n249 = Wait (ms)(milliseconds to wait=u32 150) -> ()  [unwired: 1 out]
                          }
                        }
                        n250 = invoke class="Library" method="Set Source Scope"(reference=w538, error in=w532, "SourceRef"=w535, "Scope"=w534) -> (reference out=w537:refnum<vi>, error out=w536:errorcluster)  [unwired: 1 in, 3 out]
                        n251 = invoke class="Library" method="Save"(reference=w537, error in=w532) -> (reference out=w544:refnum<vi>, error out=w543:errorcluster)  [unwired: 2 in, 2 out]
                        n252 = Close Reference(reference=w535, error in (no error)=w536) -> ()  [unwired: 1 out]
                        n253 = property class="Library"(reference=w544, error in=w543) -> (error out=w539:errorcluster, "Name"=w542:string)  [unwired: 1 out]
                      }
                      frame True {
                      }
                    }
                    n254 = case shown="True" w504 {
                      tunnel: w503 -> [w558 w559]
                      tunnel: [w557 w559] -> w502
                      tunnel: w500 -> [w556 _]
                      frame False {
                        n255 = Build Array (concatenate)(w558, w556) -> (w557:string[])
                      }
                      frame True {
                      }
                    }
                    n256 = Not Equal?(x=w512, y=w496) -> (x != y?=w509:bool)
                  }
                  n257 = Bundle(w478) -> (w477:cluster{refnum<vi>[]})  [unwired: 1 in]
                  n258 = Or Array Elements(Boolean array=w484) -> (logical OR=w483:bool)
                }
                n259 = Or Array Elements(Boolean array=w461) -> ()  [unwired: 1 out]
              }
              frame True {
                n260 = disable-structure shown="Disabled" {
                  disable-tunnel: w567 -> [w587 _]
                  disable-tunnel: w566 -> [w584 _]
                  disable-tunnel: [w581 _] -> _
                  disable-tunnel: w565 -> [w580 _]
                  disable-tunnel: w564 -> [w579 _]
                  disable-tunnel: w563 -> [w578 _]
                  disable-tunnel: [w573 _] -> w562
                  disable-tunnel: w561 -> [w571 _]
                  disable-tunnel: [w569 _] -> w560
                  frame Disabled {
                    w569 = "Clone:UpdateIcon"
                    # "The VI should not be owned by a library, only add it to the project"
                    n261 = property class="ProjectItem"(reference=w571) -> (reference out=w570:refnum<vi>, "Type String"=w568:string)  [unwired: 1 in, 1 out]
                    n262 = invoke class="VI" method="Save.Instrument"(reference=w587, error in=w580, "Path to saved file"=w579, "Save a Copy"=TRUE) -> (error out=w585:errorcluster)  [unwired: 2 in, 5 out]
                    n263 = Open VI Reference(application reference (local)=w584, vi path=w579, options=2, error in (no error)=w585) -> (vi reference=w582:refnum<vi>, error out=w572:errorcluster)  [unwired: 2 in]
                    n264 = Build Array(w582) -> (w581:refnum<vi>[])
                    n265 = case shown="Default" w568 {
                      tunnel: w579 -> [w596 w608]
                      tunnel: [w589 w607] -> w573
                      tunnel: w572 -> [w598 w604]
                      tunnel: w570 -> [w601 w602]
                      frame Default {
                        n266 = property class="ProjectItem"(reference=w601, error in=w598) -> (error out=w599:errorcluster, "Project"=w600:refnum<vi>)  [unwired: 1 out]
                        n267 = property class="Project"(reference=w600, error in=w599) -> (reference out=w588:refnum<vi>, error out=w595:errorcluster, "My Computer"=w597:refnum<vi>)
                        n268 = invoke class="TargetItem" method="AddFile"(reference=w597, error in=w595, "Path"=w596) -> (reference out=w591:refnum<vi>, error out=w593:errorcluster, "AddFile"=w594:refnum<vi>)  [unwired: 1 in, 1 out]
                        n269 = Close Reference(reference=w594, error in (no error)=w593) -> (error out=w592:errorcluster)
                        n270 = Close Reference(reference=w591, error in (no error)=w592) -> (error out=w590:errorcluster)
                        n271 = Close Reference(reference=w588, error in (no error)=w590) -> (error out=w589:errorcluster)
                      }
                      frame "Folder" {
                        n272 = property class="ProjectItem"(reference=w602, error in=w604) -> (error out=w603:errorcluster, "Connected to Disk"=w606:path)  [unwired: 1 out]
                        n273 = Empty String/Path?(string/path=w606) -> (empty?=w605:bool)
                        n274 = case shown="True" w605 {
                          tunnel: w608 -> [_ w615]
                          tunnel: [w609 w612] -> w607
                          tunnel: w603 -> [w609 w611]
                          tunnel: w602 -> [_ w610]
                          frame False {
                          }
                          frame True {
                            n275 = invoke class="ProjectItem" method="AddFile"(reference=w610, error in=w611, "Path"=w615) -> (error out=w613:errorcluster, "AddFile"=w614:refnum<vi>)  [unwired: 1 in, 2 out]
                            n276 = stacked-sequence {
                              tunnel: [w616] -> w612
                              tunnel: w613 -> [w616]
                              frame #0 {
                                n277 = Wait (ms)(milliseconds to wait=u32 150) -> ()  [unwired: 1 out]
                              }
                            }
                            n278 = Close Reference(reference=w614, error in (no error)=w612) -> ()  [unwired: 1 out]
                          }
                        }
                      }
                    }
                    n279 = Strip Path(path=w579) -> (name=w577:string)  [unwired: 1 out]
                    n280 = Strip Path(path=w578) -> (name=w576:string)  [unwired: 1 out]
                    n281 = Equal?(x=w577, y=w576) -> (x = y?=w575:bool)
                    n282 = Select(t="Done", s=w575, f=w569) -> ()  [unwired: 1 out]
                  }
                  frame Enabled {
                  }
                }
              }
            }
            n283 = Bundle By Name(cluster=w445, "FileBackups"=w450, "NewViRefs"=w441) -> (w447:T2)
          }
          frame "Clone:NewLibraryReplaceControlsAndVIs" {
            n284 = Unbundle By Name(w620) -> ("CopyToTheseClasses"=w619:refnum<vi>[])
            n285 = Unbundle By Name(w620) -> ("NewViRefs"=w618:cluster{refnum<vi>[]}[], "OrgViLibName"=w625:string, "OrgLibFolder"=w626:path, "OrgClassPathMemberData"=w624:path)
            n286 = for {
              tunnel: w626 -> [w634]
              tunnel: w625 -> [w633]
              tunnel: w624 -> [w632]
              tunnel: w619 -> [w629]
              shift-right: [w630] -> w622
              shift-left: w623 -> [w631]
              tunnel: w618 -> [w628] mode=indexing
              n287 = Unbundle(w628) -> (w627:refnum<vi>[])
              n288 = for {
                tunnel: w627 -> [w635] mode=indexing
                tunnel: w629 -> [w649] mode=indexing
                tunnel: w634 -> [w651]
                tunnel: w633 -> [w650]
                shift-right: [w638] -> w630
                shift-left: w631 -> [w648]
                tunnel: w632 -> [w640]
                n289 = property class="Library"(reference=w649, error in=w648) -> (error out=w645:errorcluster, "Name"=w646:string, "Path"=w637:path)  [unwired: 1 out]
                n290 = Strip Path(path=w637) -> (stripped path=w647:path)  [unwired: 1 out]
                n291 = call <resource>:"GOOP300_FindFilesToExchange.vi"("OldClassName(Prefix or suffix for some VIs)"=w650, "OldFolderPath"=w651, "NewFolderPath"=w647, "NewClassName(Prefix or suffix for some VIs)"=w646) -> ("OldFiles"=w644:path[], "NewFileArray"=w643:path[])  [unwired: 14 in]
                n292 = call <resource>:"Scripting_ReplaceVisAndControls.vi"("ViRef"=w635, "OldVIsAndControls"=w644, "NewVIsAndControls"=w643, "error in (no error)"=w645) -> ("error out"=w639:errorcluster)  [unwired: 14 in, 1 out]
                n293 = Build Array(w640) -> (w642:path[])
                n294 = call <vilib>:"Get File Extension.vi"("file"=w637) -> ("lowercase file extension"=w636:string)  [unwired: 6 in, 4 out]
                n295 = Build Array(w637) -> (w641:path[])
                n296 = case shown="Default" w636 {
                  tunnel: w642 -> [_ w657]
                  tunnel: w641 -> [_ w656]
                  tunnel: w635 -> [_ w655]
                  tunnel: w639 -> [w652 w654]
                  tunnel: [w652 w653] -> w638
                  frame "lvlib" {
                  }
                  frame Default {
                    n297 = call <resource>:"Scripting_ReplaceVisAndControls.vi"("ViRef"=w655, "OldVIsAndControls"=w657, "NewVIsAndControls"=w656, "error in (no error)"=w654) -> ("error out"=w653:errorcluster)  [unwired: 14 in, 1 out]
                  }
                }
              }
            }
          }
          frame "Clone:UpdateIcon" {
            n298 = Unbundle By Name(w660) -> ("CopyToTheseClasses"=w659:refnum<vi>[], "Scope"=w658:T5)
            n299 = Unbundle By Name(w660) -> ("VIRef"=w664:refnum<vi>[], "NewViRefs"=w665:cluster{refnum<vi>[]}[])
            n300 = for {
              tunnel: w665 -> [w669] mode=indexing
              tunnel: w664 -> [w667] mode=indexing
              tunnel: w659 -> [w670]
              shift-right: [w671] -> w662
              shift-left: w663 -> [w672]
              tunnel: w658 -> [w666] mode=indexing
              n301 = Unbundle(w669) -> (w668:refnum<vi>[])
              n302 = property class="VI"(reference=w667) -> ("Path"=w674:path)  [unwired: 1 in, 2 out]
              n303 = call <resource>:"GDSLvIcon_AnalyseViIcon.vi"("ViRef/LvCLassRef/LvLibRef/ViPath/2D_Image"=w667, "error in (no error)"=w672) -> ("BodyBkColor"=w675:u32, "error out"=w676:errorcluster)  [unwired: 5 in, 11 out]
              n304 = call <vilib>:"Get File Extension.vi"("file"=w674) -> ("filename without extension"=w673:string)  [unwired: 6 in, 4 out]
              n305 = for {
                tunnel: w668 -> [w683] mode=indexing
                shift-right: [w689] -> w671
                shift-left: w676 -> [w690]
                tunnel: w670 -> [w688]
                tunnel: w675 -> [w684]
                tunnel: w673 -> [w680]
                tunnel: w666 -> [w677]
                i -> [w687]
                n306 = property class="VI"(reference=w683) -> ("Path"=w682:path)  [unwired: 1 in, 2 out]
                n307 = Index Array(array=w688, index=w687) -> (element=w678:refnum<vi>)
                n308 = Not A Number/Path/Refnum?(number/path/refnum=w678) -> (NaN/Path/Refnum?=w686:bool)
                n309 = call <vilib>:"Get File Extension.vi"("file"=w682) -> ("filename without extension"=w681:string)  [unwired: 6 in, 4 out]
                n310 = Not Equal?(x=w680, y=w681) -> (x != y?=w679:bool)
                n311 = Compound Arithmetic op=OR(w679, w686) -> (w685:bool)
                n312 = case shown="False" w685 {
                  tunnel: w683 -> [w709 w763]
                  tunnel: w690 -> [w711 w762]
                  tunnel: [w712 w761] -> w689
                  tunnel: w684 -> [w716 _]
                  tunnel: [_ w760] -> _
                  tunnel: w678 -> [w707 _]
                  tunnel: w677 -> [w702 _]
                  frame False {
                    # "Take header from New Class Liberary\nBody Body from current VI\nReplace CurrentBody color with New\nClass Library Body color"
                    n313 = To More Specific Class(target class=refnum<vi> refnum ("Class Refnum In"), reference=w707) -> (specific class reference=w714:refnum<vi>, error out=w713:errorcluster)  [unwired: 1 in]
                    n314 = case shown="No Error" w713 {
                      tunnel: w714 -> [w734 _]
                      tunnel: w707 -> [_ w756]
                      tunnel: [w726 w749] -> w706
                      tunnel: [w725 w748] -> w705
                      tunnel: [w733 w750] -> w704
                      tunnel: [w723 w751] -> w703
                      tunnel: w702 -> [w720 _]
                      frame No Error {
                        n315 = property class="LVClassLibrary"(reference=w734) -> ("Member Data"=w732:refnum<vi>)  [unwired: 1 in, 2 out]
                        n316 = call <resource>:"GDSLvClass_ReadClassColors.vi"("Library Refnum"=w734) -> ("LvClassIconSettings"=w730:T6, "LvClassIconSettingsFound"=w729:bool)  [unwired: 13 in, 4 out]
                        n317 = Unbundle By Name(w730) -> ("Frame"=w722:u32, "Frame thickness"=w721:u8, "ColorPublic"=w719:u32, "ColorProtected"=w717:u32, "ColorPrivate"=w718:u32)
                        n318 = call <resource>:"GDSLvIcon_AnalyseViIcon.vi"("ViRef/LvCLassRef/LvLibRef/ViPath/2D_Image"=w732) -> ("FrameColor"=w728:u32, "FrameThickness(1)"=w727:u32, "HeaderIcon"=w733:u8[][], "BodyBkColor"=w724:u32, "error out"=w731:errorcluster)  [unwired: 6 in, 8 out]
                        n319 = case shown="True" w729 {
                          tunnel: w728 -> [w737 _]
                          tunnel: w727 -> [w736 _]
                          tunnel: [w737 w744] -> w726
                          tunnel: [w736 w743] -> w725
                          tunnel: w724 -> [w735 _]
                          tunnel: [w735 w740] -> w723
                          tunnel: w722 -> [_ w744]
                          tunnel: w721 -> [_ w743]
                          tunnel: w720 -> [_ w742]
                          tunnel: w719 -> [_ w741]
                          tunnel: w718 -> [_ w739]
                          tunnel: w717 -> [_ w738]
                          frame False {
                          }
                          frame True {
                            n320 = case shown="\"public\", Default" w742 {
                              tunnel: w741 -> [_ _ w747]
                              tunnel: [w745 w746 w747] -> w740
                              tunnel: w739 -> [w745 _ _]
                              tunnel: w738 -> [_ w746 _]
                              frame "private" {
                              }
                              frame "protected" {
                              }
                              frame "public", Default {
                              }
                            }
                          }
                        }
                        n321 = Close Reference(reference=w732, error in (no error)=w731) -> ()  [unwired: 1 out]
                      }
                      frame Error {
                        n322 = invoke class="Library" method="Get All Descendents"(reference=w756, "Type"="VI") -> ("All Descendents"=w757:refnum<vi>[])  [unwired: 5 in, 6 out]
                        n323 = Index Array(array=w757) -> (element=w758:refnum<vi>)  [unwired: 1 in]
                        n324 = property class="ProjectItem"(reference=w758) -> (error out=w754:errorcluster, "Reference"=w755:refnum<vi>)  [unwired: 1 in, 1 out]
                        n325 = call <resource>:"GDSLvIcon_AnalyseViIcon.vi"("ViRef/LvCLassRef/LvLibRef/ViPath/2D_Image"=w755, "error in (no error)"=w754) -> ("FrameColor"=w749:u32, "FrameThickness(1)"=w748:u32, "HeaderIcon"=w750:u8[][], "BodyBkColor"=w751:u32, "error out"=w753:errorcluster)  [unwired: 5 in, 8 out]
                        n326 = Close Reference(reference=w757, error in (no error)=w753) -> (error out=w752:errorcluster)
                        n327 = Close Reference(reference=w755, error in (no error)=w752) -> ()  [unwired: 1 out]
                      }
                    }
                    n328 = call <resource>:"GDSLvIcon_AnalyseViIcon.vi"("ViRef/LvCLassRef/LvLibRef/ViPath/2D_Image"=w709, "error in (no error)"=w711) -> ("BodyIcon"=w708:u8[][], "error out"=w710:errorcluster)  [unwired: 5 in, 11 out]
                    n329 = call <resource>:"GDSLvIcon_ReplaceIconColor.vi"("IconIn"=w708, "OldColor"=w716, "NewColor"=w703, "error in (no error)"=w710) -> ("IconOut"=w694:u8[][], "error out"=w696:errorcluster)  [unwired: 14 in]
                    n330 = call <resource>:"GDSLvIcon_CreateIconPicture.vi"("FrameColor"=w706, "FrameThickness(1)"=w705, "HeaderIconIn"=w704, "BodyIconIn"=w694, "error in (no error)"=w696) -> ("WholeIconOut"=w699:u8[][], "error out"=w695:errorcluster)  [unwired: 9 in, 4 out]
                    n331 = Reshape Array(w699, 1024 ("dimension size")) -> (w697:u8[])
                    n332 = Bundle By Name(cluster=T4 {"image type"=0, "image depth"=8, "image"=[], "mask"=[], "colors"=[], "Rectangle"={"left"=0, "top"=0, "right"=32, "bottom"=32}} ("image data"), "image"=w697) -> (w700:T4)
                    n333 = invoke class="VI" method="VI Icon.Set from Image Data"(reference=w709, error in=w695, "ImageData"=w700) -> (reference out=w692:refnum<vi>, error out=w693:errorcluster)  [unwired: 3 in, 4 out]
                    n334 = call <resource>:"Scripting_SaveVi.vi"("ForceResaving(False)"=TRUE, "error in (no error)"=w693, "VIRefToSaveIn"=w692) -> ("error out"=w712:errorcluster)  [unwired: 7 in, 1 out]
                  }
                  frame True {
                    n335 = stacked-sequence {
                      tunnel: w763 -> [w764]
                      tunnel: w762 -> [w766]
                      tunnel: [w765] -> w761
                      tunnel: [w764] -> w760
                      frame #0 {
                        n336 = call <resource>:"GDSIconEditor_CreateVIIcon.vi"("ViRef(IgnoreIfNotWired)"=w764, "error in (no error)"=w766) -> ("error out"=w765:errorcluster)  [unwired: 9 in]
                      }
                    }
                  }
                }
              }
            }
          }
          frame "Done", "Error", Default {
            n337 = Unbundle By Name(w769) -> ("OpenAfter"=w768:bool, "CopyToTheseClasses"=w767:refnum<vi>[])
            n338 = Unbundle By Name(w769) -> ("FileBackups"=w774:string[], "VIRef"=w776:refnum<vi>[], "NewViRefs"=w782:cluster{refnum<vi>[]}[], "VIOwner"=w781:refnum<vi>, "AppRef"=w779:refnum<vi>)
            n339 = for {
              tunnel: w782 -> [w800] mode=indexing
              shift-right: [w802] -> w778
              shift-left: w772 -> [w803]
              tunnel: w768 -> [w801]
              n340 = Unbundle(w800) -> (w799:refnum<vi>[])
              n341 = for {
                tunnel: w801 -> [w805]
                shift-right: [w810] -> w802
                shift-left: w803 -> [w811]
                tunnel: w799 -> [w804] mode=indexing
                n342 = invoke class="VI" method="Save.Instrument"(reference=w804, error in=w811) -> (reference out=w809:refnum<vi>, error out=w807:errorcluster)  [unwired: 4 in, 4 out]
                n343 = case shown="False" w805 {
                  tunnel: w809 -> [w813 w818]
                  tunnel: [w812 w816] -> w808
                  tunnel: w807 -> [w812 w815]
                  tunnel: [w813 w814] -> w806
                  frame False {
                  }
                  frame True {
                    n344 = property class="VI"(reference=w818, error in=w815, "Front Panel.Open"=TRUE ("Front Panel Window:Open")) -> (reference out=w814:refnum<vi>, error out=w816:errorcluster)
                  }
                }
                n345 = Close Reference(reference=w806, error in (no error)=w808) -> (error out=w810:errorcluster)
              }
            }
            n346 = Close Reference(reference=w767) -> ()  [unwired: 1 in, 1 out]
            n347 = Empty Array?(array=w774) -> (empty?=w775:bool)
            n348 = Close Reference(reference=w776, error in (no error)=w778) -> (error out=w777:errorcluster)
            n349 = Close Reference(reference=w781, error in (no error)=w777) -> (error out=w780:errorcluster)
            n350 = Array Size(array=w774) -> (size(s)=w773:i32)
            n351 = Close Reference(reference=w779, error in (no error)=w780) -> (error out=w771:errorcluster)
            n352 = case shown="False" w775 {
              tunnel: w773 -> [w786 _]
              tunnel: w770 -> [w785 _]
              tunnel: w771 -> [_ _]
              frame False {
                n353 = case shown="1" w786 {
                  tunnel: ["%d file has been overwritten.\nA backup of this could be found here:\n%s" ("message") "%d files have been overwritten.\nA backup of these could be found here:\n%s" ("message")] -> w787
                  frame 1 {
                  }
                  frame 2, Default {
                  }
                }
                n354 = Format Into String(format string=w787, w786, w785) -> (resulting string=w784:string)  [unwired: 2 in, 1 out]
                n355 = stacked-sequence {
                  tunnel: w784 -> [w790]
                  frame #0 {
                    n356 = feedback #1() -> (w788:bool)  [unwired: 1 in]
                    n357 = case shown="False" w788 {
                      selector: w788 -> [_ w796]
                      tunnel: w790 -> [w795 _]
                      tunnel: [w791 w796] -> w789
                      frame False {
                        n358 = Two Button Dialog(message=w795, 1:"OK (Don't show in future)" ("F button name (\"Cancel\")"), 2:"OK" ("T button name (\"OK\")")) -> (T button?=w792:bool)
                        n359 = Not(x=w792) -> (.not. x?=w791:bool)
                      }
                      frame True {
                      }
                    }
                    n360 = feedback-in #1(w789) -> ()
                  }
                }
              }
              frame True {
              }
            }
          }
        }
        n361 = Equal?(x=w23, y="Exit") -> (x = y?=w26:bool)
        n362 = Select(t="Error", s=w25, f=w23) -> (s? t:f=w24:string)
      }
    }
    frame Error {
    }
  }
  "error out" <- w8
  n363 = stacked-sequence {
    tunnel: w10 -> [w820]
    tunnel: [w822] -> w9
    frame #0 {
      w821 = TRUE ("Visible")
      n364 = Unbundle By Name(w820) -> ("Cancel"=w822:bool)
      n365 = property on="_ViPathAlreadyExists" class="Bool (strict)"("Visible"=w821) -> ()  [unwired: 2 in, 2 out]
      n366 = property on="_CloneMethodClasses" class="LstBox (strict)"("Visible"=w821) -> ()  [unwired: 2 in, 2 out]
    }
  }
  "Cancelled" <- w9
